vi "LED_Set.vi"(8 "error in (no error)":errorcluster caption="错误输入（无错误）", 10 "Result":bool[](array[boolean]), 11 "VISA资源名称":refnum<visa-resource-name>) -> (0 "error out":errorcluster caption="错误输出", 1 "Close CMD":string, 2 "Open CMD":string, 3 "VISA资源名称输出":refnum<visa-resource-name>)   [LabVIEW 2018]
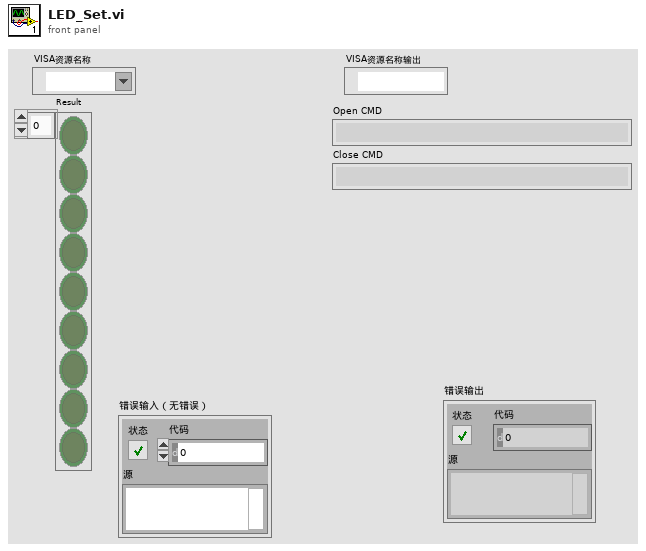
[diagram p1: front panel]
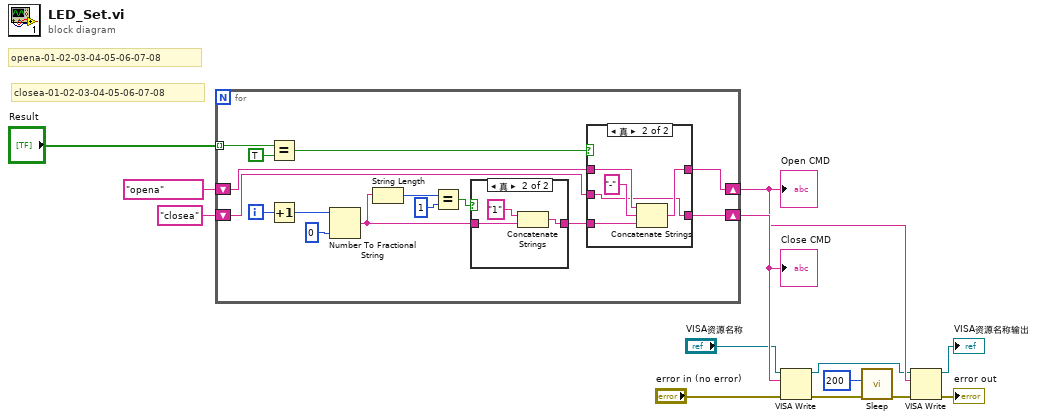
[diagram p0: block diagram]
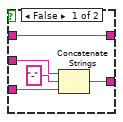
[diagram p2: hidden frame]
diagram:
  # "closea-01-02-03-04-05-06-07-08"
  # "opena-01-02-03-04-05-06-07-08"
  n1 = for {
    tunnel: "Result" -> [w26] mode=indexing
    shift-right: [w27] -> w9
    shift-left: "opena" -> [w28]
    shift-right: [w14] -> w10
    shift-left: "closea" -> [w15]
    i -> [w23]
    n2 = Equal?(x=w26, y=TRUE) -> (x = y?=w16:bool)
    n3 = Increment(x=w23) -> (x+1=w22:i32)
    n4 = Number To Fractional String(number=w22, precision (6)=i16 0 ("精度(6)")) -> (F-format string=w18:string)  [unwired: 2 in]
    n5 = String Length(string=w18) -> (length=w21:i32)
    n6 = Equal?(x=w21, y=1) -> (x = y?=w19:bool)
    n7 = case shown="真" w19 {
      tunnel: w18 -> [w39 w41]
      tunnel: [w39 w40] -> w17
      frame False {
      }
      frame True {
        n8 = Concatenate Strings("1" ("字符串"), w41) -> (w40:string)
      }
    }
    n9 = case shown="真" w16 {
      tunnel: w28 -> [w33 w38]
      tunnel: [w33 w37] -> w27
      tunnel: w17 -> [w30 w35]
      tunnel: w15 -> [w31 w34]
      tunnel: [w29 w34] -> w14
      frame False {
        n10 = Concatenate Strings(w31, "-" ("字符串"), w30) -> (w29:string)
      }
      frame True {
        n11 = Concatenate Strings(w38, "-" ("字符串"), w35) -> (w37:string)
      }
    }
  }
  "Open CMD" <- w9
  "Close CMD" <- w10
  n12 = VISA Write(VISA resource name="VISA资源名称", write buffer=w10, error in (no error)="error in (no error)") -> (VISA resource name out=w3:refnum<visa-resource-name>, error out=w5:errorcluster)  [unwired: 1 out]
  n13 = call "Sleep.vi"("error in (no error)"=w5, "等待时间（毫秒）"=u32 200) -> ("error out"=w4:errorcluster)  [unwired: 9 in]
  n14 = VISA Write(VISA resource name=w3, write buffer=w9, error in (no error)=w4) -> (VISA resource name out=→"VISA资源名称输出":refnum<visa-resource-name>, error out=→"error out":errorcluster)  [unwired: 1 out]
